vi "tearDown.vi"(8 "error in (no error)":errorcluster, 11 "reference in":refnum<class "csm-ini-variable-addon.lvclass">) -> (0 "error out":errorcluster, 3 "reference out":refnum<class "csm-ini-variable-addon.lvclass">)   [LabVIEW 2017, in "csm-ini-variable-addon.lvclass"]
doc: "tearDown runs after the test method has completed. Use this method to clean up any operations or references that were opened by setUp or the test method. Unit tests should be independent of other unit tests so this VI should ensure that the next test can run in a 'clean' test environment."
uses:
  csm-ini-variable-addon.lvclass
  csm-ini-variable-addon.lvclass/csm-ini-variable-addon.ctl
  INI-Static-Variable-Support/INI-Static-Variable-Support.lvlib
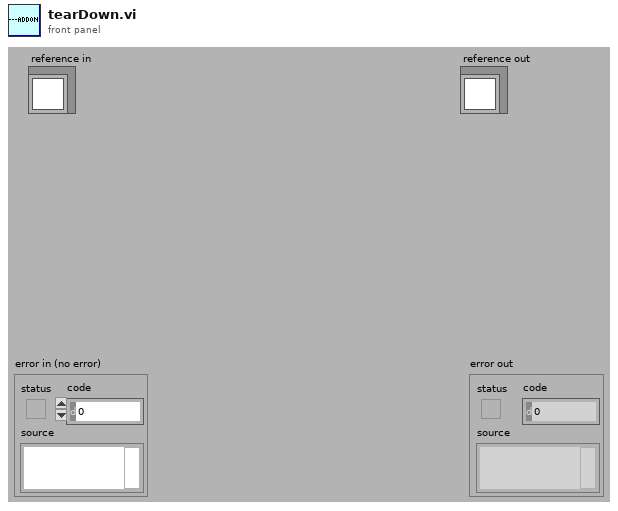
[diagram p1: front panel]
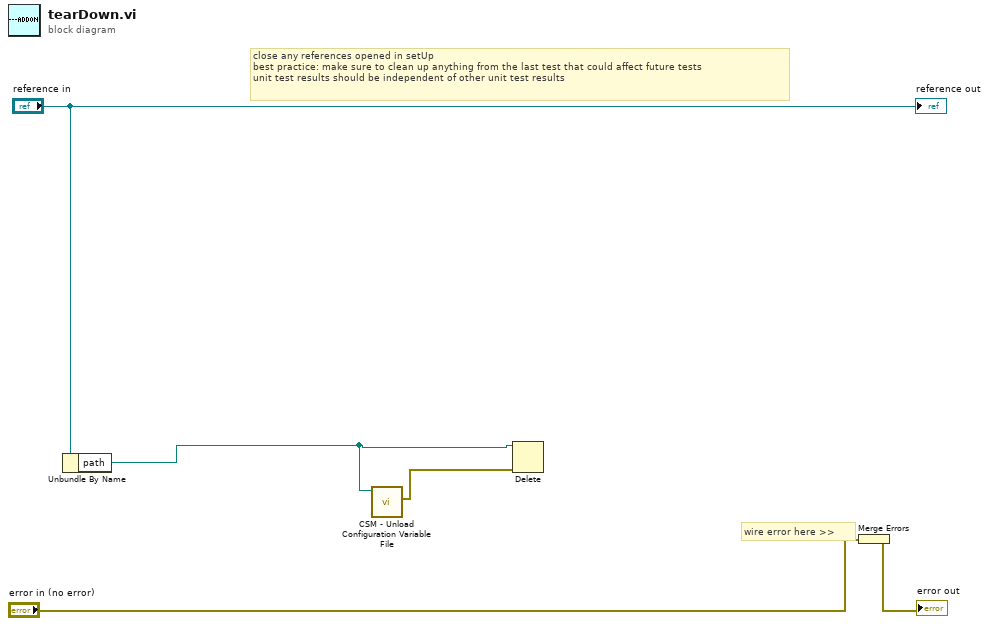
[diagram p0: block diagram]
diagram:
  # "wire error here >>"
  # "close any references opened in setUp\nbest practice: make sure to clean up anything from the last test that could affect future tests\nunit test results should be independent of other unit test results"
  n1 = Unbundle By Name("reference in") -> ("path"=w1:path)
  n2 = call "CSM - Unload Configuration Variable File.vi"("Path"=w1) -> ("error out"=w2:errorcluster)  [unwired: 8 in]
  n3 = Delete(path (use dialog)=w1, error in=w2) -> ()  [unwired: 3 in, 3 out]
  n4 = Merge Errors("error in (no error)") -> (→"error out":errorcluster)
  "reference out" <- "reference in"
